vi "ArmGetPosition.vi"() -> (1 "ExtendPostion":dbl, 2 "LiftPostion":dbl)   [LabVIEW 2023]
doc: "Get current position\n\nOutput:\n--RotatePosition -- Double -- Degrees\n--LiftPosition -- Double -- Degrees\n--ExtendPosition -- Double -- Inches"
uses:
  ArmGlobal.vi
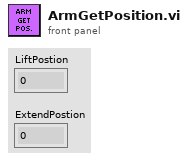
[diagram p1: front panel]
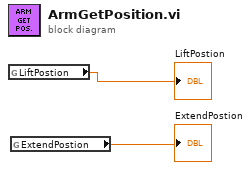
[diagram p0: block diagram]
diagram:
  n1 = global read "ArmGlobal.vi" "LiftPostion"() -> (→"LiftPostion":dbl)
  n2 = global read "ArmGlobal.vi" "ExtendPostion"() -> (→"ExtendPostion":dbl)
